vi "Test_serializerINI.vi"(8 "error in (no error)":errorcluster) -> (0 "error out":errorcluster)   [LabVIEW 2013]
uses:
  source/Serializer.INI/Serializer.PlainText.INI.lvclass
  <vilib>/addons/_JKI Toolkits/Caraya/classes/Assert/Assert Equal Value_Variant.vi
  <vilib>/addons/_JKI Toolkits/Caraya/classes/Assert/Assert Not Error.vi
  <vilib>/addons/_JKI Toolkits/Caraya/classes/Assert/Assert Equal Value and Type_Variant.vi
  <vilib>/addons/_JKI Toolkits/Caraya/classes/Assert/Assert Almost Equal_Float.vi
  source/Serializer/Serializer.lvclass
  <vilib>/addons/_JKI Toolkits/Caraya/classes/Test/Test.lvclass
  <vilib>/addons/_JKI Toolkits/Caraya/classes/Assert/Assert.lvclass
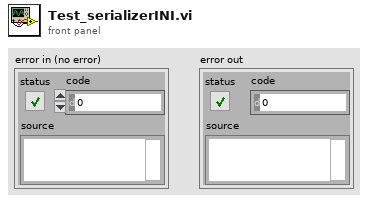
[diagram p1: front panel]
types:
  T1 = cluster{"numeric":i32, "Array":errorcluster[][], "Embedded Cluster":cluster{"EmbeddedArray":errorcluster[]}, "Boolean":bool, "String":string, "myPath":path, "myStringArray":string[][], "myNumericsArray":dbl[]}
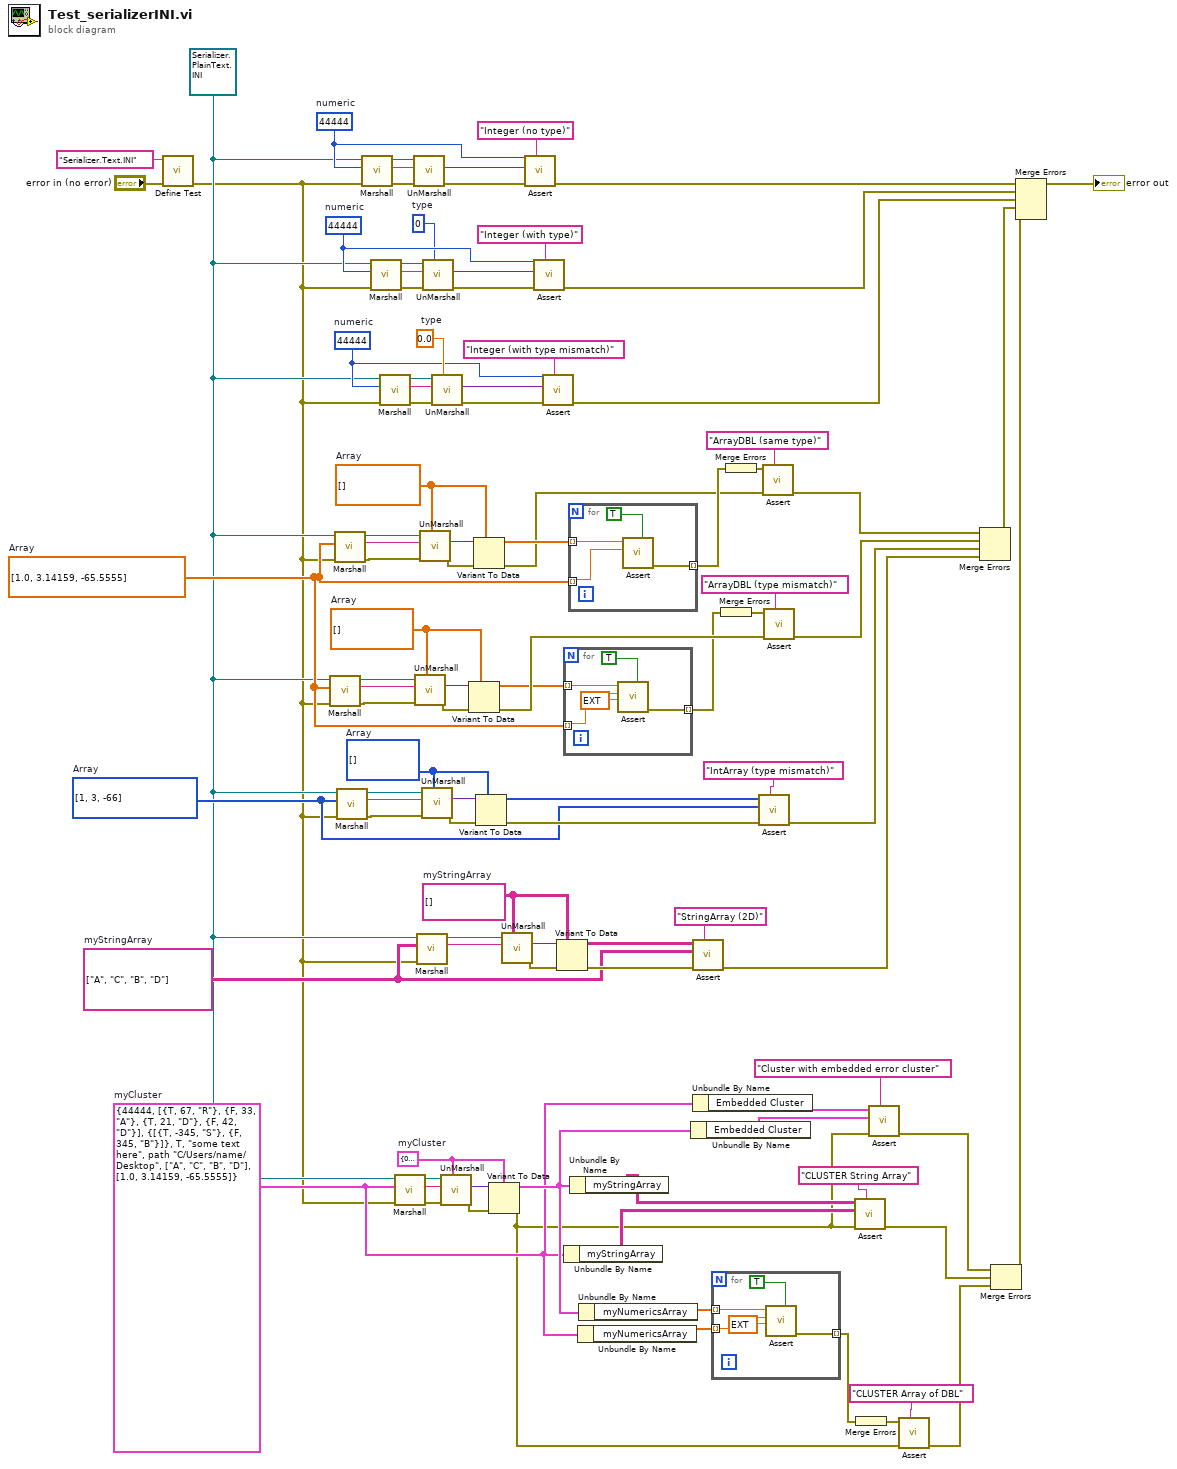
[diagram p0: block diagram]
diagram:
  w29 = i64[] [1, 3, -66]  # Array
  w36 = i16[] []  # Array
  w46 = sgl[] []  # Array
  w66 = 0.0  # type
  w59 = 44444  # numeric
  w70 = 0  # type
  w77 = 44444  # numeric
  w78 = 44444  # numeric
  w21 = refnum<class "Serializer.PlainText.INI.lvclass"> refnum ("OpenSerializer.lvlib:Serializer.PlainText.INI.lvclass")
  w90 = string[][] []  # myStringArray
  w24 = string[][] [["A", "C"], ["B", "D"]]  # myStringArray
  w97 = dbl[] []  # Array
  w27 = dbl[] [1.0, 3.14159, -65.5555]  # Array
  w12 = T1 {"numeric"=0, "Array"=[], "Embedded Cluster"={"EmbeddedArray"=[]}, "Boolean"=FALSE, "String"="", "myPath"=path "", "myStringArray"=[], "myNumericsArray"=[]}  # myCluster
  w87 = T1 {"numeric"=44444, "Array"=[[{"status"=TRUE, "code"=67, "source"="R"}, {"status"=FALSE, "code"=33, "source"="A"}, {"status"=TRUE, "code"=21, "source"="D"}, {"status"=FALSE, "code"=42, "source"="D"}]], "Embedded Cluster"={"EmbeddedArray"=[{"status"=TRUE, "code"=-345, "source"="S"}, {"status"=FALSE, "code"=345, "source"="B"}]}, "Boolean"=TRUE, "String"="some text here", "myPath"=path "C:/Users/name/Desktop", "myStringArray"=[["A", "C"], ["B", "D"]], "myNumericsArray"=[1.0, 3.14159, -65.5555]}  # myCluster
  n1 = call <vilib>:"Define Test.vi"("error in (no error)"="error in (no error)", "Label (VI Title)"="Serializer.Text.INI") -> ("error out"=w20:errorcluster)  [unwired: 9 in]
  n2 = call "Marshall.vi"("error in (no error)"=w20, "Variant"=w27, "Serializer in"=w21) -> ("error out"=w51:errorcluster, "String"=w47:string, "Serializer out"=w45:refnum<class "Serializer.PlainText.INI.lvclass">)  [unwired: 6 in]
  n3 = call "Marshall.vi"("error in (no error)"=w20, "Variant"=w27, "Serializer in"=w21) -> ("error out"=w54:errorcluster, "String"=w96:string, "Serializer out"=w98:refnum<class "Serializer.PlainText.INI.lvclass">)  [unwired: 6 in]
  n4 = call "Marshall.vi"("error in (no error)"=w20, "Variant"=w29, "Serializer in"=w21) -> ("error out"=w33:errorcluster, "String"=w35:string, "Serializer out"=w37:refnum<class "Serializer.PlainText.INI.lvclass">)  [unwired: 6 in]
  n5 = call "Marshall.vi"("error in (no error)"=w20, "Variant"=w78, "Serializer in"=w21) -> ("error out"=w84:errorcluster, "String"=w83:string, "Serializer out"=w82:refnum<class "Serializer.PlainText.INI.lvclass">)  [unwired: 6 in]
  n6 = call "Marshall.vi"("error in (no error)"=w20, "Variant"=w77, "Serializer in"=w21) -> ("error out"=w71:errorcluster, "String"=w72:string, "Serializer out"=w73:refnum<class "Serializer.PlainText.INI.lvclass">)  [unwired: 6 in]
  n7 = call "Marshall.vi"("error in (no error)"=w20, "Variant"=w59, "Serializer in"=w21) -> ("error out"=w65:errorcluster, "String"=w64:string, "Serializer out"=w63:refnum<class "Serializer.PlainText.INI.lvclass">)  [unwired: 6 in]
  n8 = call "Marshall.vi"("error in (no error)"=w20, "Variant"=w87, "Serializer in"=w21) -> ("error out"=w13:errorcluster, "String"=w95:string, "Serializer out"=w101:refnum<class "Serializer.PlainText.INI.lvclass">)  [unwired: 6 in]
  n9 = call "UnMarshall.vi"("error in (no error)"=w84, "String"=w83, "Serializer in"=w82) -> ("error out"=w79:errorcluster, "Variant"=w81:variant)  [unwired: 6 in, 1 out]
  n10 = call "UnMarshall.vi"("Type"=w46, "error in (no error)"=w51, "String"=w47, "Serializer in"=w45) -> ("error out"=w44:errorcluster, "Variant"=w43:variant)  [unwired: 5 in, 1 out]
  n11 = call "Marshall.vi"("error in (no error)"=w20, "Variant"=w24, "Serializer in"=w21) -> ("String"=w94:string, "Serializer out"=w93:refnum<class "Serializer.PlainText.INI.lvclass">)  [unwired: 6 in, 1 out]
  n12 = call "UnMarshall.vi"("Type"=w97, "error in (no error)"=w54, "String"=w96, "Serializer in"=w98) -> ("error out"=w99:errorcluster, "Variant"=w100:variant)  [unwired: 5 in, 1 out]
  n13 = call "UnMarshall.vi"("Type"=w36, "error in (no error)"=w33, "String"=w35, "Serializer in"=w37) -> ("error out"=w38:errorcluster, "Variant"=w39:variant)  [unwired: 5 in, 1 out]
  n14 = call "UnMarshall.vi"("Type"=w70, "error in (no error)"=w71, "String"=w72, "Serializer in"=w73) -> ("error out"=w76:errorcluster, "Variant"=w74:variant)  [unwired: 5 in, 1 out]
  n15 = call "UnMarshall.vi"("Type"=w66, "error in (no error)"=w65, "String"=w64, "Serializer in"=w63) -> ("error out"=w60:errorcluster, "Variant"=w62:variant)  [unwired: 5 in, 1 out]
  n16 = call "UnMarshall.vi"("Type"=w12, "error in (no error)"=w13, "String"=w95, "Serializer in"=w101) -> ("error out"=w14:errorcluster, "Variant"=w102:variant)  [unwired: 5 in, 1 out]
  n17 = Variant To Data(error in=w44, type=w46, Variant=w43) -> (data=w28:sgl[], error out=w50:errorcluster)
  n18 = Variant To Data(error in=w99, type=w97, Variant=w100) -> (data=w89:dbl[], error out=w55:errorcluster)
  n19 = Variant To Data(error in=w38, type=w36, Variant=w39) -> (data=w30:i16[], error out=w34:errorcluster)
  n20 = Variant To Data(error in=w14, type=w12, Variant=w102) -> (data=w88:T1, error out=w4:errorcluster)
  n21 = call "UnMarshall.vi"("Type"=w90, "String"=w94, "Serializer in"=w93) -> ("error out"=w92:errorcluster, "Variant"=w91:variant)  [unwired: 6 in, 1 out]
  n22 = call-poly <vilib>:"Assert.vi"("Label"="Integer (no type)" ("Label (VI Title)"), "error in (no error)"=w79, "Y"=w81, "X"=w78) -> ("error out"=w68:errorcluster)  [unwired: 7 in]
  n23 = call-poly <vilib>:"Assert.vi"("Label"="Integer (with type)" ("Label (VI Title)"), "error in (no error)"=w76, "Y"=w74, "X"=w77) -> ("error out"=w69:errorcluster)  [unwired: 7 in]
  n24 = call-poly <vilib>:"Assert.vi"("Label"="Integer (with type mismatch)" ("Label (VI Title)"), "error in (no error)"=w60, "Y"=w62, "X"=w59) -> ("error out"=w58:errorcluster)  [unwired: 7 in]
  n25 = Variant To Data(error in=w92, type=w90, Variant=w91) -> (data=w25:string[][], error out=w26:errorcluster)
  n26 = for {
    tunnel: w28 -> [w107] mode=indexing
    tunnel: w27 -> [w106] mode=indexing
    tunnel: [w104] -> w48 mode=indexing
    n27 = call-poly <vilib>:"Assert.vi"("Assert Only? (F)"=TRUE, "Tolerance"=ext 0.00001, "Y"=w106, "X"=w107) -> ("error out"=w104:errorcluster)  [unwired: 7 in]
  }
  n28 = Unbundle By Name(w87) -> ("myStringArray"=w5:string[][])
  n29 = for {
    tunnel: w89 -> [w111] mode=indexing
    tunnel: w27 -> [w110] mode=indexing
    tunnel: [w108] -> w57 mode=indexing
    n30 = call-poly <vilib>:"Assert.vi"("Assert Only? (F)"=TRUE, "Y"=w110, "X"=w111) -> ("error out"=w108:errorcluster)  [unwired: 8 in]
  }
  n31 = Unbundle By Name(w88) -> ("myStringArray"=w6:string[][])
  n32 = Unbundle By Name(w87) -> ("myNumericsArray"=w15:dbl[])
  n33 = Unbundle By Name(w88) -> ("myNumericsArray"=w16:dbl[])
  n34 = Unbundle By Name(w88) -> ("Embedded Cluster"=w9:cluster{"EmbeddedArray":errorcluster[]})
  n35 = call-poly <vilib>:"Assert.vi"("Label"="StringArray (2D)" ("Label (VI Title)"), "error in (no error)"=w26, "Y"=w24, "X"=w25) -> ("error out"=w22:errorcluster)  [unwired: 7 in]
  n36 = Unbundle By Name(w87) -> ("Embedded Cluster"=w10:cluster{"EmbeddedArray":errorcluster[]})
  n37 = for {
    tunnel: w16 -> [w116] mode=indexing
    tunnel: w15 -> [w115] mode=indexing
    tunnel: [w113] -> w19 mode=indexing
    n38 = call-poly <vilib>:"Assert.vi"("Assert Only? (F)"=TRUE, "Tolerance"=ext 0.00001, "Y"=w115, "X"=w116) -> ("error out"=w113:errorcluster)  [unwired: 7 in]
  }
  n39 = Merge Errors(w48) -> (w49:errorcluster)
  n40 = Merge Errors(w57) -> (w56:errorcluster)
  n41 = call-poly <vilib>:"Assert.vi"("Label"="IntArray (type mismatch)" ("Label (VI Title)"), "error in (no error)"=w34, "Y"=w29, "X"=w30) -> ("error out"=w31:errorcluster)  [unwired: 7 in]
  n42 = call-poly <vilib>:"Assert.vi"("Label"="ArrayDBL (same type)" ("Label (VI Title)"), "error in (no error)"=w55, "Not Error?"=w56) -> ("error out"=w41:errorcluster)  [unwired: 8 in]
  n43 = call-poly <vilib>:"Assert.vi"("Label"="ArrayDBL (type mismatch)" ("Label (VI Title)"), "error in (no error)"=w50, "Not Error?"=w49) -> ("error out"=w42:errorcluster)  [unwired: 8 in]
  n44 = call-poly <vilib>:"Assert.vi"("Label"="CLUSTER String Array" ("Label (VI Title)"), "error in (no error)"=w4, "Y"=w5, "X"=w6) -> ("error out"=w3:errorcluster)  [unwired: 7 in]
  n45 = Merge Errors(w19) -> (w18:errorcluster)
  n46 = call-poly <vilib>:"Assert.vi"("Label"="Cluster with embedded error cluster" ("Label (VI Title)"), "error in (no error)"=w4, "Y"=w9, "X"=w10) -> ("error out"=w7:errorcluster)  [unwired: 7 in]
  n47 = call-poly <vilib>:"Assert.vi"("Label"="CLUSTER Array of DBL" ("Label (VI Title)"), "error in (no error)"=w4, "Not Error?"=w18) -> ("error out"=w11:errorcluster)  [unwired: 8 in]
  n48 = Merge Errors(w41, w42, w31, w22) -> (w40:errorcluster)
  n49 = Merge Errors(w7, w3, w11) -> (w1:errorcluster)
  n50 = Merge Errors(w68, w69, w58, w40, w1) -> (→"error out":errorcluster)
